vi "Return Weight.vi"(8 "error in":errorcluster, 10 "Weight Number":i32, 11 "GrabberTool in":refnum<class "GrabberTool Class.lvclass">) -> (0 "error out":errorcluster, 3 "GrabberTool out":refnum<class "GrabberTool Class.lvclass">)   [LabVIEW 2011, in "GrabberTool Class.lvclass"]
uses:
  GrabberTool Class.lvclass
  Config Manager Class/Type Definitions/Named Position.ctl
  Config Manager Class/Type Definitions/Part Type.ctl
  Config Manager Class/Type Definitions/Offset.ctl
  WorkTable Class/WorkTable Class.lvclass
  Vec3d Class/Vec3d Class.lvclass
  Config Manager Class/Read Geometry Definition 3D.vi
  Config Manager Class/Config Manager Class.lvclass
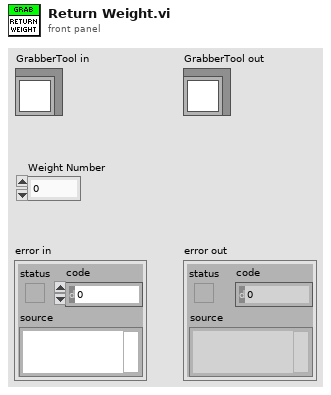
[diagram p1: front panel]
types:
  T1 = typedef "Named Position.ctl" = enum16{"home", "module_chuck_0", "module_chuck_1", "module_chuck_2", "module_chuck_3", "module_chuck_4", "glue_reservoir_chuck", "stamp_tool_chuck", "weight_tool_chuck", "needle_calibration", "tool_rack_pos_0_in", "tool_rack_pos_0_out", "tool_rack_pos_1_in", "tool_rack_pos_1_out", "tool_rack_pos_2_in", "tool_rack_pos_2_out", "front_load_position", "grabber_start_pos", "between_chuck_0_and_1", "between_chuck_2_and_3"}
  T2 = typedef "Part Type.ctl" = enum16{"BBM", "HDI", "BARE HDI", "GLUERESERVOIR", "STAMP_1", "STAMP_2", "STAMP_3", "STAMP_4", "STAMP_5", "WEIGHT_1", "WEIGHT_2", "WEIGHT_3", "WEIGHT_4", "WEIGHT_5", "WEIGHT_6", "WEIGHT_7", "WEIGHT_8", "PICKER_TOOL", "GRABER_TOOL"}
  T3 = typedef "Offset.ctl" = enum16{"needle_offset", "tool_holder_offset"}
  T4 = typedef "Worktable_Weights.ctl" = cluster{"Weight Slots":cluster{"Weight State":enum16{"Empty", "Populated"}, "Weight Type":T5, "Location/Orientation":T6}[], "Vacuum Channel":i32}
  T5 = typedef "Weight Type.ctl" = enum16{"Weight 1", "Weight 2", "Weight 3", "Weight 4", "Weight 5", "Weight 6", "Weight 7", "Weight 8"}
  T6 = typedef "Position_Orientation.ctl" = cluster{"Center":refnum<class "Vec3d Class.lvclass">, "Orientation":refnum<class "Orient3d Class.lvclass">}
  T7 = cluster{"Weight State":enum16{"Empty", "Populated"}, "Weight Type":T5, "Location/Orientation":T6}[]
  T8 = cluster{"Weight State":enum16{"Empty", "Populated"}, "Weight Type":T5, "Location/Orientation":T6}
  T9 = typedef "Gluing Parameters.ctl" = cluster{"Safe Grabber Pickup":dbl, "Safe Grabber Lift":dbl, "Glue Resevoir Wait Time":dbl, "Glue BM Wait Time ":dbl, "Placed Weight X-Move":dbl}
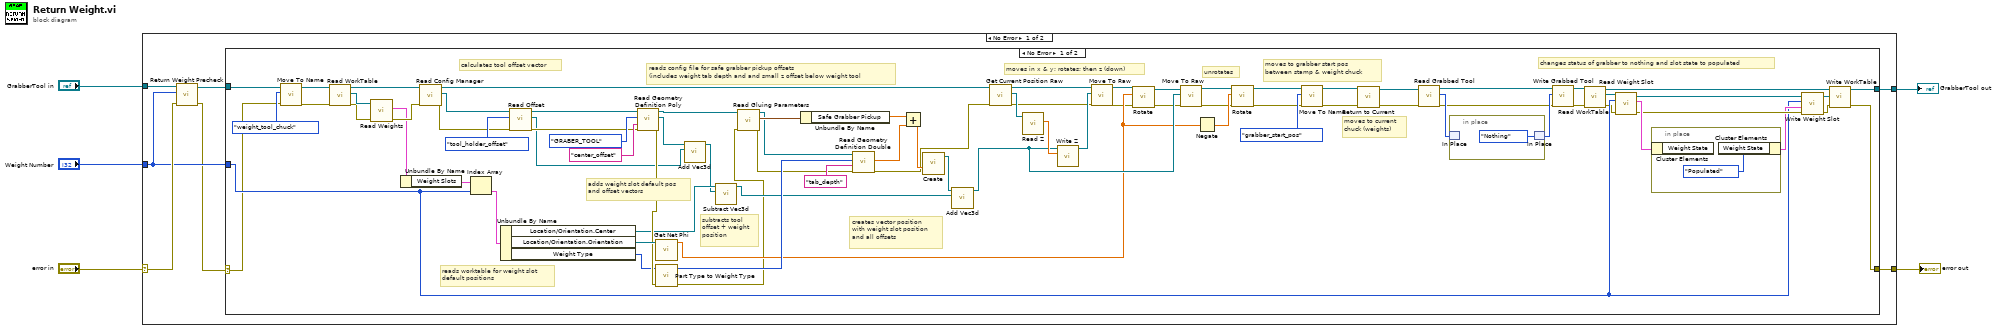
[diagram p0: block diagram]
diagram:
  n1 = case shown="No Error" "error in" {
    selector: "error in" -> [w11 w96]
    tunnel: [w6 w96] -> w4
    tunnel: [w7 w95] -> w2
    tunnel: "GrabberTool in" -> [w12 w95]
    tunnel: "Weight Number" -> [w10 _]
    frame No Error {
      n2 = call "Return Weight Precheck.vi"("error in"=w11, "Weight Number"=w10, "GrabberTool in"=w12) -> ("error out"=w8:errorcluster, "GrabberTool out"=w9:refnum<class "GrabberTool Class.lvclass">)  [unwired: 7 in]
      n3 = case shown="No Error" w8 {
        selector: w8 -> [w13 w93]
        tunnel: w10 -> [w34 _]
        tunnel: w9 -> [w90 w94]
        tunnel: [w32 w94] -> w7
        tunnel: [w31 w93] -> w6
        frame No Error {
          # "moves to current\nchuck (weights)"
          # "changes status of grabber to nothing and slot state to populated"
          # "moves to grabber start pos\nbetween stamp & weight chuck"
          # "unrotates"
          # "moves in x & y; rotates; then z (down)"
          # "subtracts tool\noffset + weight\nposition"
          # "creates vector position\nwith weight slot position\nand all offsets"
          # "reads config file for safe grabber pickup offsets\n(includes weight tab depth and and small z offset below weight tool"
          # "adds weight slot default pos\nand offset vectors"
          # "reads worktable for weight slot\ndefault positions"
          # "calculates tool offset vector"
          n4 = call-dynamic "Move To Name.vi"("error in"=w13, "Destination"=Named_Position."weight_tool_chuck", "Gantry in"=w90) -> ("error out"=w14:errorcluster, "Gantry out"=w88:refnum<class "GrabberTool Class.lvclass">)  [unwired: 7 in]
          n5 = call-dynamic "Read WorkTable.vi"("error in"=w14, "Gantry Class in"=w88) -> ("error out"=w15:errorcluster, "WorkTable Class.lvclass"=w74:refnum<class "WorkTable Class.lvclass">, "Gantry Class out"=w75:refnum<class "GrabberTool Class.lvclass">)  [unwired: 7 in]
          n6 = call-dynamic "Read Weights.vi"("error in (no error)"=w15, "WorkTable Class in"=w74) -> ("error out"=w87:errorcluster, "Weights"=w86:T4)  [unwired: 7 in, 1 out]
          n7 = Unbundle By Name(w86) -> ("Weight Slots"=w85:T7)
          n8 = call-dynamic "Read Config Manager.vi"("error in"=w87, "Gantry in"=w75) -> ("error out"=w78:errorcluster, "Config Manager"=w82:refnum<class "Config Manager Class.lvclass">, "Gantry out"=w59:refnum<class "GrabberTool Class.lvclass">)  [unwired: 7 in]
          n9 = Index Array(array=w85, index=w34) -> (element=w84:T8)
          n10 = Unbundle By Name(w84) -> ("Location/Orientation.Center"=w70:refnum<class "Vec3d Class.lvclass">, "Location/Orientation.Orientation"=w79:refnum<class "Orient3d Class.lvclass">, "Weight Type"=w35:T5)
          n11 = call "Read Offset.vi"("error in"=w78, "Offset"=Offset."tool_holder_offset", "Config Manager in"=w82) -> ("error out"=w77:errorcluster, "Vec3d out"=w71:refnum<class "Vec3d Class.lvclass">)  [unwired: 6 in, 1 out]
          n12 = call-poly "Read Geometry Definition Poly.vi"("error in"=w77, "Feature"="center_offset", "Part Type"=Part_Type."GRABER_TOOL", "Config Manager in"=w82) -> ("error out"=w76:errorcluster, "Feature Coordinates"=w72:refnum<class "Vec3d Class.lvclass">, "Config Manager out"=w73:refnum<class "Config Manager Class.lvclass">)  [unwired: 5 in]
          n13 = call "Get Net Phi.vi"("Orient3d"=w79) -> ("phi(deg)"=w47:dbl)  [unwired: 8 in, 2 out]
          n14 = call "Part Type to Weight Type.vi"("error in"=w76, "Weight Type"=w35) -> ("error out"=w16:errorcluster, "Part Type"=w63:T2)  [unwired: 8 in]
          n15 = call-dynamic "Add Vec3d.vi"(10:"Vec3d Class in"=w71, 11:"Vec3d Class in"=w72) -> ("Vec3d Class out"=w69:refnum<class "Vec3d Class.lvclass">)  [unwired: 8 in, 1 out]
          n16 = call "Subtract Vec3d.vi"("Vec3d in 2"=w69, "Vec3d in 1"=w70) -> ("Vec3d Class out"=w62:refnum<class "Vec3d Class.lvclass">)  [unwired: 8 in, 1 out]
          n17 = call "Read Gluing Parameters.vi"("error in (no error)"=w16, "Config Manager Class in"=w73) -> ("error out"=w17:errorcluster, "Gluing Parameters"=w68:T9, "Config Manager Class out"=w65:refnum<class "Config Manager Class.lvclass">)  [unwired: 7 in]
          n18 = Unbundle By Name(w68) -> ("Safe Grabber Pickup"=w67:dbl)
          n19 = call "Read Geometry Definition Double.vi"("error in"=w17, "Feature"="tab_depth", "Part Type"=w63, "Config Manager in"=w65) -> ("error out"=w18:errorcluster, "Geometry Definition"=w66:dbl)  [unwired: 5 in, 1 out]
          n20 = Add(x=w67, y=w66) -> (x+y=w61:dbl)
          n21 = call "Create.vi"("Z"=w61) -> ("Vec3d Class out"=w60:refnum<class "Vec3d Class.lvclass">)  [unwired: 9 in, 1 out]
          n22 = call-dynamic "Add Vec3d.vi"(10:"Vec3d Class in"=w62, 11:"Vec3d Class in"=w60) -> ("Vec3d Class out"=w54:refnum<class "Vec3d Class.lvclass">)  [unwired: 8 in, 1 out]
          n23 = call-dynamic "Get Current Position Raw.vi"("error in"=w18, "Gantry in"=w59) -> ("error out"=w19:errorcluster, "Vec3d Class out"=w58:refnum<class "Vec3d Class.lvclass">, "Gantry out"=w56:refnum<class "GrabberTool Class.lvclass">)  [unwired: 7 in]
          n24 = call-dynamic "Read Z.vi"("Vec3d Class in"=w58) -> ("Z"=w57:dbl)  [unwired: 8 in, 2 out]
          n25 = call-dynamic "Write Z.vi"("Z"=w57, "Vec3d Class in"=w54) -> ("Vec3d Class out"=w55:refnum<class "Vec3d Class.lvclass">)  [unwired: 8 in, 1 out]
          n26 = call-dynamic "Move To Raw.vi"("error in"=w19, "Destination"=w55, "Gantry in"=w56) -> ("error out"=w20:errorcluster, "Gantry out"=w53:refnum<class "GrabberTool Class.lvclass">)  [unwired: 7 in]
          n27 = call-dynamic "Rotate.vi"("error in"=w20, "distance(deg)"=w47, "Gantry in"=w53) -> ("error out"=w21:errorcluster, "Gantry out"=w52:refnum<class "GrabberTool Class.lvclass">)  [unwired: 7 in]
          n28 = call-dynamic "Move To Raw.vi"("error in"=w21, "Destination"=w54, "Gantry in"=w52) -> ("error out"=w22:errorcluster, "Gantry out"=w50:refnum<class "GrabberTool Class.lvclass">)  [unwired: 7 in]
          n29 = Negate(x=w47) -> (-x=w48:dbl)
          n30 = call-dynamic "Rotate.vi"("error in"=w22, "distance(deg)"=w48, "Gantry in"=w50) -> ("error out"=w27:errorcluster, "Gantry out"=w49:refnum<class "GrabberTool Class.lvclass">)  [unwired: 7 in]
          n31 = call-dynamic "Move To Name.vi"("error in"=w27, "Destination"=Named_Position."grabber_start_pos", "Gantry in"=w49) -> ("error out"=w23:errorcluster, "Gantry out"=w26:refnum<class "GrabberTool Class.lvclass">)  [unwired: 7 in]
          n32 = call-dynamic "Return to Current.vi"("error in"=w23, "Gantry in"=w26) -> ("error out"=w24:errorcluster, "Gantry out"=w25:refnum<class "GrabberTool Class.lvclass">)  [unwired: 8 in]
          n33 = call "Read Grabbed Tool.vi"("error in (no error)"=w24, "GrabberTool Class in"=w25) -> ("error out"=w43:errorcluster, "Grabbed Tool"=w46:enum16{"Weight Tool", "Stamp Tool", "Nothing"}, "GrabberTool Class out"=w44:refnum<class "GrabberTool Class.lvclass">)  [unwired: 7 in]
          n34 = in-place {
            n35 = in-place-match #1(w46) -> ()  [unwired: 1 out]
            n36 = in-place-match #1(enum16{"Weight Tool", "Stamp Tool", "Nothing"}."Nothing" ("Grabbed Tool")) -> (w45:enum16{"Weight Tool", "Stamp Tool", "Nothing"})
          }
          n37 = call "Write Grabbed Tool.vi"("error in (no error)"=w43, "Grabbed Tool"=w45, "GrabberTool Class in"=w44) -> ("error out"=w28:errorcluster, "GrabberTool Class out"=w41:refnum<class "GrabberTool Class.lvclass">)  [unwired: 7 in]
          n38 = call-dynamic "Read WorkTable.vi"("error in"=w28, "Gantry Class in"=w41) -> ("error out"=w29:errorcluster, "WorkTable Class.lvclass"=w40:refnum<class "WorkTable Class.lvclass">, "Gantry Class out"=w42:refnum<class "GrabberTool Class.lvclass">)  [unwired: 7 in]
          n39 = call "Read Weight Slot.vi"("error in (no error)"=w29, "weight slot"=w34, "WorkTable Class in"=w40) -> ("error out"=w37:errorcluster, "Weight Slot"=w39:T8, "WorkTable Class out"=w38:refnum<class "WorkTable Class.lvclass">)  [unwired: 6 in]
          n40 = in-place {
            n41 = in-place-cluster #2(w39) -> ()  [unwired: 1 out]
            n42 = in-place-cluster #2("Weight State"=enum16{"Empty", "Populated", "Used"}."Populated" ("Stamp State")) -> (w36:T8)
          }
          n43 = call "Write Weight Slot.vi"("error in (no error)"=w37, "Weight Slot"=w36, "weight slot"=w34, "WorkTable Class in"=w38) -> ("error out"=w30:errorcluster, "WorkTable Class out"=w33:refnum<class "WorkTable Class.lvclass">)  [unwired: 6 in]
          n44 = call-dynamic "Write WorkTable.vi"("error in (no error)"=w30, "WorkTable Class.lvclass"=w33, "Gantry Class in"=w42) -> ("error out"=w31:errorcluster, "Gantry Class out"=w32:refnum<class "GrabberTool Class.lvclass">)  [unwired: 7 in]
        }
        frame Error {
        }
      }
    }
    frame Error {
    }
  }
  "error out" <- w4
  "GrabberTool out" <- w2
